vi "State Machine 1.vi"() -> ()   [LabVIEW 2015]
panel:
  in  "Stop Button":bool
  out "RED":bool
  out "YELLOW":bool
  out "GREEN":bool
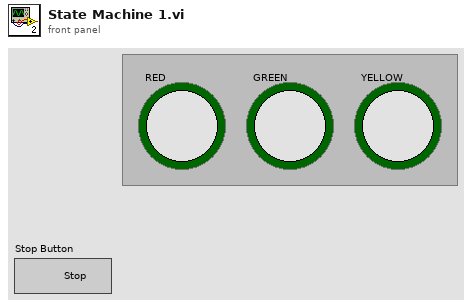
[diagram p1: front panel]
types:
  T1 = enum16{"START", "INITIALIZE", "RED", "GREEN", "YELLOW", "CONTINUE", "STOP"}
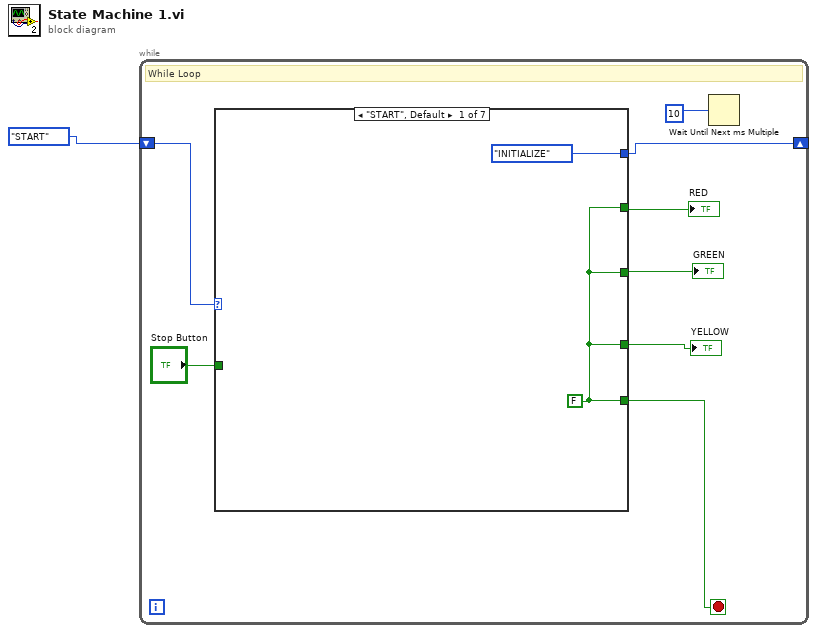
[diagram p0: block diagram]
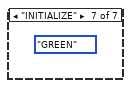
[diagram p7: hidden frame]
diagram:
  n1 = while {
    shift-right: [w8] -> _
    shift-left: T1."START" -> [w9]
    stop <- w7 stop-if-true
    # "While Loop"
    n2 = case shown="\"START\", Default" w9 {
      tunnel: [T1."INITIALIZE" _ _ _ _ _ _] -> w8
      tunnel: [w10 _ _ _ _ _ _] -> w6
      tunnel: [w10 _ _ _ _ _ _] -> w4
      tunnel: [w10 _ _ _ _ _ _] -> w5
      tunnel: [w10 _ _ _ _ _ _] -> w7
      tunnel: "Stop Button" -> [_ _ _ _ _ _ _]
      frame "START", Default {
        w10 = FALSE
      }
      frame "RED" {
      }
      frame "GREEN" {
      }
      frame "YELLOW" {
      }
      frame "CONTINUE" {
      }
      frame "STOP" {
      }
      frame "INITIALIZE" {
        (unwired) T1."GREEN"
      }
    }
    "GREEN" <- w5
    "RED" <- w6
    "YELLOW" <- w4
    n3 = Wait Until Next ms Multiple(millisecond multiple=10) -> ()  [unwired: 1 out]
  }
